vi "References Updated.vi"(6 "Dependencies":bool[](array[boolean]), 8 "error in":errorcluster, 9 "Modules Types":T1[](array[typedef]), 10 "Modules":refnum<vi>[](array[refnum]), 11 "Application Instance":refnum<vi>) -> (0 "error out":errorcluster)   [LabVIEW 2019, in "Panther Dashboard.lvlib"]
doc: "DQMH Module and Event references has being updated\n_____\nCreated using DQMH Event Scripter 6.1.0.128."
uses:
  Panther Dashboard.lvlib
  Module type--enum.ctl
  References Updated Argument--cluster.ctl
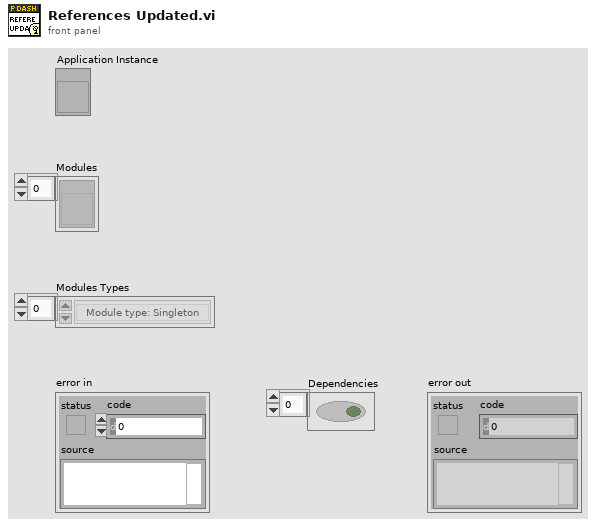
[diagram p1: front panel]
types:
  T1 = typedef "Panther Dashboard.lvlib/Module type--enum.ctl" = enum16{"Module type: Singleton", "Module type: Cloneable"}
  T2 = typedef "Panther Dashboard.lvlib/References Updated Argument--cluster.ctl" = cluster{"Modules":refnum<vi>[], "Modules Types":T1[], "Application Instance":refnum<vi>, "Dependencies":bool[]}
  T3 = typedef "Panther Dashboard.lvlib/Broadcast Events--cluster.ctl" = cluster{"Module Did Init":refnum<user-event>, "Status Updated":refnum<user-event>, "Error Reported":refnum<user-event>, "Module Did Stop":refnum<user-event>, "Update Module Execution Status":refnum<user-event>, "References Updated":refnum<user-event>, "Projects Updated":refnum<user-event>, "Targets Updated":refnum<user-event>, "Progress updated":refnum<user-event>, "Scale Updated":refnum<user-event>, "Connector Pane Updated":refnum<user-event>, "Documentation Updated":refnum<user-event>, "Module Type Updated":refnum<user-event>, "Theme Updated":refnum<user-event>, "Project Description Updated":refnum<user-event>}
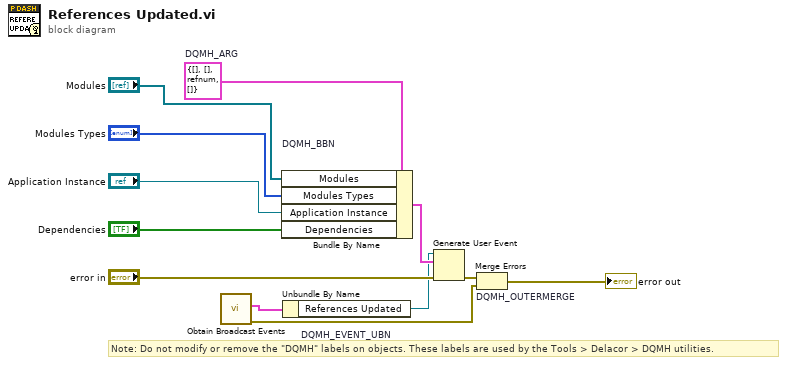
[diagram p0: block diagram]
diagram:
  w6 = T2 {"Modules"=[], "Modules Types"=[], "Application Instance"=refnum, "Dependencies"=[]}  # DQMH_ARG
  # "Note: Do not modify or remove the \"DQMH\" labels on objects. These labels are used by the Tools > Delacor > DQMH utilities."
  n1 = call "Obtain Broadcast Events.vi"() -> ("error out"=w9:errorcluster, "Panther Dashboard Broadcast Events"=w5:T3)  [unwired: 10 in]
  n2 = Bundle By Name "DQMH_BBN"(cluster=w6, "Modules"="Modules", "Modules Types"="Modules Types", "Application Instance"="Application Instance", "Dependencies"="Dependencies") -> (w8:T2)
  n3 = Unbundle By Name "DQMH_EVENT_UBN"(w5) -> ("References Updated"=w7:refnum<user-event>)
  n4 = Generate User Event(user event=w7, event data cluster=w8, error in="error in") -> (error out=w10:errorcluster)  [unwired: 1 in, 1 out]
  n5 = Merge Errors "DQMH_OUTERMERGE"(w10, w9) -> (→"error out":errorcluster)
